vi "StartCaller.vi"   [LabVIEW 2018]
uses:
  Counter.lvclass/Counter.lvclass
  C:/Program Files (x86)/National Instruments/LabVIEW 2018/vi.lib/ActorFramework/Actor/Actor.lvclass
  <vilib>/ActorFramework/Actor/Actor.lvclass
panel:
  # "Start To Run"
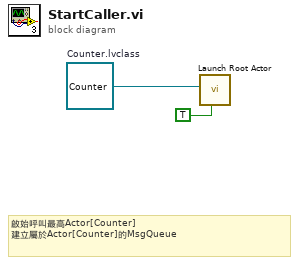
[diagram p0: block diagram]
diagram:
  w2 = refnum<class "Counter.lvclass"> refnum  # Counter.lvclass
  # "啟始呼叫最高Actor[Counter]\n建立屬於Actor[Counter]的MsgQueue"
  n1 = call <vilib>:"Launch Root Actor.vi"("Open Actor Core front panel? (F)"=TRUE, "Actor"=w2) -> ()  [unwired: 8 in, 2 out]
